vi "CalcTUR.vi"(7 "PMUConfig":T1, 8 "error in (no error)":errorcluster, 10 "Uncertainties":dbl[][][](array[numeric]) format="%#_2g", 11 "Limits":dbl[][](array[numeric])) -> (0 "error out":errorcluster, 2 "TUR":dbl[][](array[numeric]))   [LabVIEW 2014]
uses:
  typedef/PMUConfig.ctl
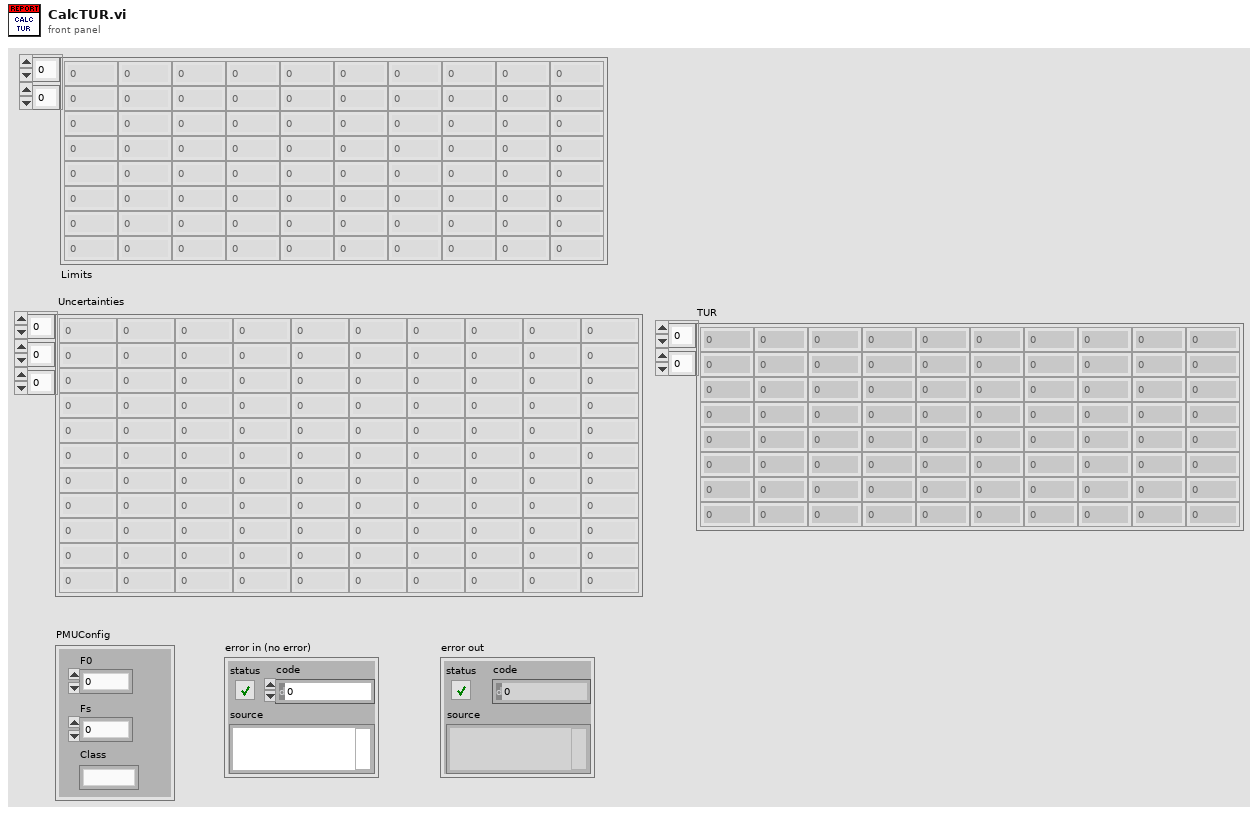
[diagram p1: front panel]
types:
  T1 = typedef "PMUConfig.ctl" = cluster{"Class":string, "Fs":dbl, "F0":dbl}
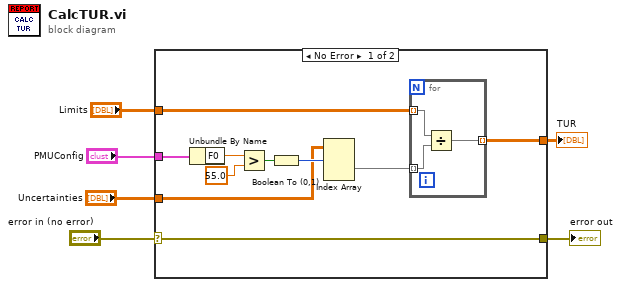
[diagram p0: block diagram]
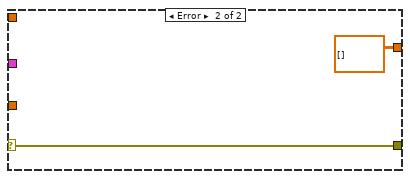
[diagram p2: hidden frame]
diagram:
  n1 = case shown="No Error" "error in (no error)" {
    selector: "error in (no error)" -> [w7 w21]
    tunnel: [w7 w21] -> w5
    tunnel: "PMUConfig" -> [w16 _]
    tunnel: "Uncertainties" -> [w11 _]
    tunnel: "Limits" -> [w10 _]
    tunnel: [w8 dbl[][] []] -> w1
    frame No Error {
      n2 = Unbundle By Name(w16) -> ("F0"=w15:dbl)
      n3 = Greater?(x=w15, y=55.0) -> (0:w13:bool)
      n4 = Boolean To (0,1)(Boolean=w13) -> (0, 1=w12:i16)
      n5 = Index Array(array=w11, index (dim 0)=w12) -> (element=w9:dbl[][])  [unwired: 2 in]
      n6 = for {
        tunnel: w10 -> [w19] mode=indexing
        tunnel: w9 -> [w18] mode=indexing
        tunnel: [w17] -> w8 mode=indexing
        n7 = Divide(x=w19, y=w18) -> (x/y=w17:dbl[])
      }
    }
    frame Error {
    }
  }
  "error out" <- w5
  "TUR" <- w1
